vi "Handle RESULT.vi"(8 "error in (no error)":errorcluster, 9 "Message Loop Shift Register Data":T1, 10 "WAMP Message":T16 {"Message Codes" items=["HELLO"=1, "WELCOME"=2, "ABORT"=3, "GOODBYE"=6, "ERROR"=8, "PUBLISH"=16, "PUBLISHED"=17, "SUBSCRIBE"=32, "SUBSCRIBED"=33, "UNSUBSCRIBE"=34, "UNSUBSCRIBED"=35, "EVENT"=36, "CALL"=48, "RESULT"=59, "REGISTER"=64, "REGISTERED"=65, "UNREGISTER"=66, "UNREGISTERED"=67, "INVOCATION"=68, "YIELD"=70]}, 11 "reference":refnum<class "WAMP Client.lvclass">) -> (0 "error out":errorcluster, 1 "Message Loop Shift Register Data (out)":T1, 3 "reference out":refnum<class "WAMP Client.lvclass">)   [LabVIEW 2020, in "wamplv.lvlib" / "WAMP Client.lvclass"]
uses:
  WAMP Client.lvclass
  TypeDef/WAMP Received Message.ctl
  TypeDef/WAMP Message Codes.ctl
  TypeDef/Message Loop Shift Reg Data.ctl
  TypeDef/REGISTER Request Data.ctl
  TypeDef/Success or error.ctl
  API/TypeDefs/Combined error.ctl
  API/TypeDefs/WAMP error.ctl
  API/TypeDefs/Invocation payload.ctl
  TypeDef/Publish Requests Map.ctl
  TypeDef/PUBLISH Request Data.ctl
  TypeDef/PUBLISH Result.ctl
  TypeDef/Endpoint Data.ctl
  TypeDef/CALL Request Map.ctl
  TypeDef/CALL Request Data.ctl
  API/TypeDefs/RESULT Payload.ctl
  TypeDef/SUBSCRIBE Requests Map.ctl
  TypeDef/SUBSCRIBE Request Data.ctl
  TypeDef/Subscribe Result.ctl
  TypeDef/Event Payload.ctl
  TypeDef/Subscriptions Map.ctl
  TypeDef/Subscription Details.ctl
  TypeDef/Unsubscribe Requests Map.ctl
  TypeDef/UNSUBSCRIBE Request Data.ctl
  TypeDef/UNSUBSCRIBE Result.ctl
  TypeDef/Unregister requests map.ctl
  TypeDef/Unregister request.ctl
  WAMP Client.lvclass/WAMP Client.ctl
  <vilib>/JDP Science/JSONtext/JSONtext.lvlib
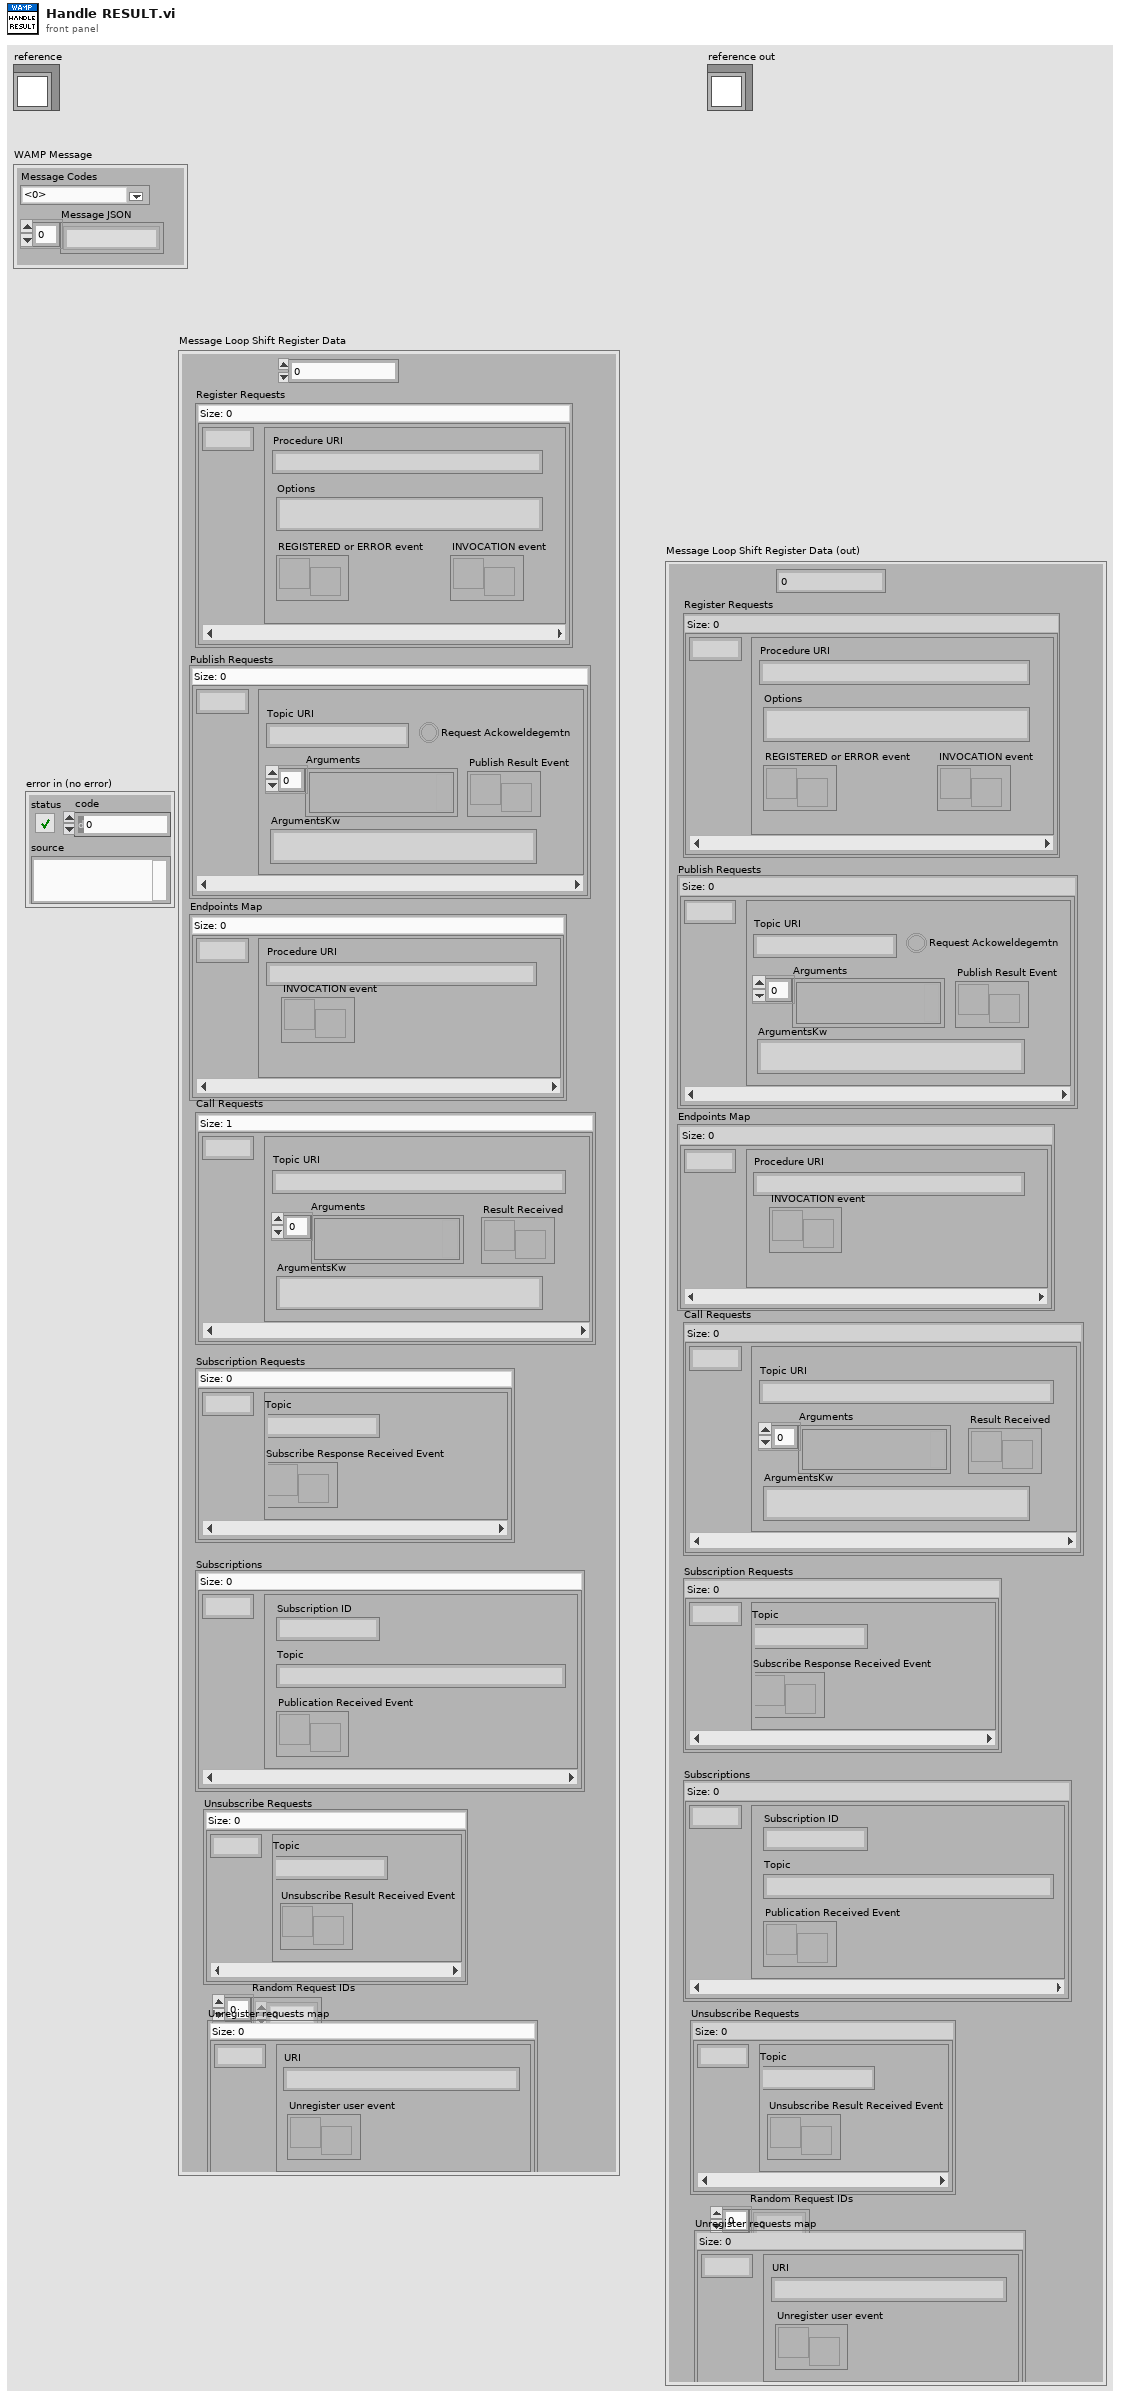
[diagram p1: front panel]
types:
  T1 = typedef "wamplv.lvlib/WAMP Client.lvclass/Message Loop Shift Reg Data.ctl" = cluster{"Last Request ID":u64, "Register Requests":map{u64, T2}, "Publish Requests":T3, "Endpoints Map":map{u64, T5}, "Call Requests":T6, "Subscription Requests":T8, "Subscriptions":T10, "Unsubscribe Requests":T12, "Random Request IDs":u64[], "Unregister requests map":T14}
  T2 = typedef "wamplv.lvlib/WAMP Client.lvclass/REGISTER Request Data.ctl" = cluster{"Procedure URI":string, "Options":string, "REGISTERED or ERROR event":refnum<user-event>, "INVOCATION event":refnum<user-event>}
  T3 = typedef "wamplv.lvlib/WAMP Client.lvclass/Publish Requests Map.ctl" = map{u64, T4}
  T4 = typedef "wamplv.lvlib/WAMP Client.lvclass/PUBLISH Request Data.ctl" = cluster{"Topic URI":string, "Arguments":variant[], "ArgumentsKw":string, "Publish Result Event":refnum<user-event>, "Request Ackoweldegemtn":bool}
  T5 = typedef "wamplv.lvlib/WAMP Client.lvclass/Endpoint Data.ctl" = cluster{"Procedure URI":string, "INVOCATION event":refnum<user-event>}
  T6 = typedef "wamplv.lvlib/WAMP Client.lvclass/CALL Request Map.ctl" = map{u64, T7}
  T7 = typedef "wamplv.lvlib/WAMP Client.lvclass/CALL Request Data.ctl" = cluster{"Topic URI":string, "Arguments":variant[], "ArgumentsKw":string, "Result Received":refnum<user-event>}
  T8 = typedef "wamplv.lvlib/WAMP Client.lvclass/SUBSCRIBE Requests Map.ctl" = map{u64, T9}
  T9 = typedef "wamplv.lvlib/WAMP Client.lvclass/SUBSCRIBE Request Data.ctl" = cluster{"Topic":string, "Subscribe Response Received Event":refnum<user-event>}
  T10 = typedef "wamplv.lvlib/WAMP Client.lvclass/Subscriptions Map.ctl" = map{u64, T11}
  T11 = typedef "wamplv.lvlib/WAMP Client.lvclass/Subscription Details.ctl" = cluster{"Subscription ID":u64, "Topic":string, "Publication Received Event":refnum<user-event>}
  T12 = typedef "wamplv.lvlib/WAMP Client.lvclass/Unsubscribe Requests Map.ctl" = map{u64, T13}
  T13 = typedef "wamplv.lvlib/WAMP Client.lvclass/UNSUBSCRIBE Request Data.ctl" = cluster{"Topic":string, "Unsubscribe Result Received Event":refnum<user-event>}
  T14 = typedef "wamplv.lvlib/WAMP Client.lvclass/Unregister requests map.ctl" = map{u64, T15}
  T15 = typedef "wamplv.lvlib/WAMP Client.lvclass/Unregister request.ctl" = cluster{"URI":string, "Unregister user event":refnum<user-event>}
  T16 = typedef "wamplv.lvlib/WAMP Client.lvclass/WAMP Received Message.ctl" = cluster{"Message JSON":string[], "Message Codes":T17}
  T17 = typedef "wamplv.lvlib/WAMP Client.lvclass/WAMP Message Codes.ctl" = u16
  T18 = typedef "wamplv.lvlib/WAMP Client.lvclass/RESULT Payload.ctl" = cluster{"Arguments Payload":string[], "ArgumentKw Payload":string, "Topic":string, "Success?":bool, "Combined Error":T19}
  T19 = typedef "wamplv.lvlib/WAMP Client.lvclass/Combined error.ctl" = cluster{"Error?":bool, "WAMP Error":T20, "Error":errorcluster}
  T20 = typedef "wamplv.lvlib/WAMP Client.lvclass/WAMP error.ctl" = cluster{"Details":string, "ArgumentKw Payload":string, "Error?":bool, "Error URI":string, "Arguments Payload":string[]}
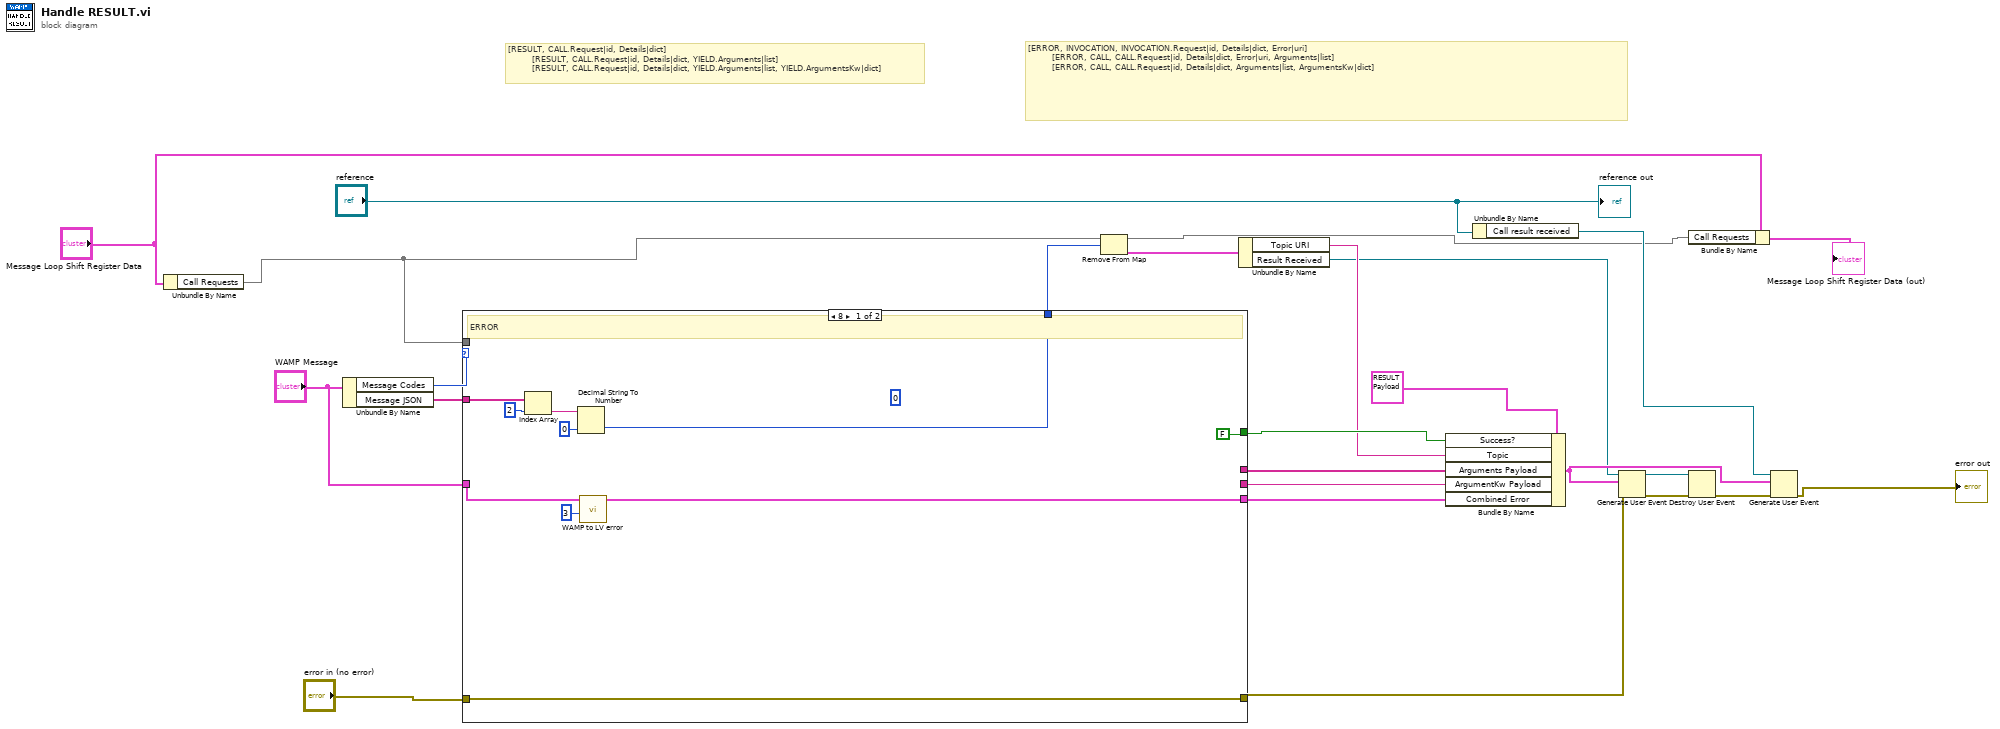
[diagram p0: block diagram]
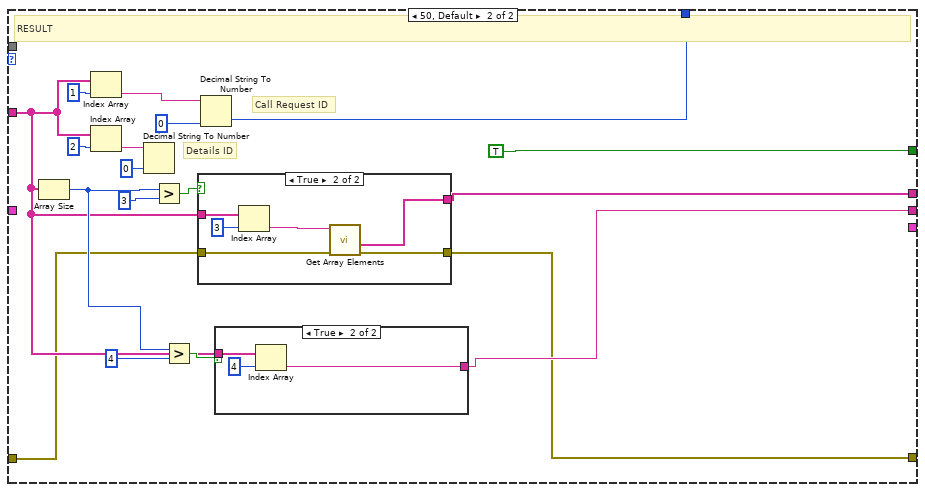
[diagram p2: hidden frame]
diagram:
  # "[ERROR, INVOCATION, INVOCATION.Request|id, Details|dict, Error|uri]\n        [ERROR, CALL, CALL.Request|id, Details|dict, Error|uri, Arguments|list]\n        [ERROR, CALL, CALL.Request|id, Details|dict, Arguments|list, ArgumentsKw|dict]"
  # "[RESULT, CALL.Request|id, Details|dict]\n        [RESULT, CALL.Request|id, Details|dict, YIELD.Arguments|list]\n        [RESULT, CALL.Request|id, Details|dict, YIELD.Arguments|list, YIELD.ArgumentsKw|dict]"
  n1 = Unbundle By Name("Message Loop Shift Register Data") -> ("Call Requests"=w7:T6)
  n2 = Unbundle By Name("WAMP Message") -> ("Message Codes"=w22:T17, "Message JSON"=w21:string[])
  n3 = case shown="8" w22 {
    tunnel: w21 -> [w31 w40]
    tunnel: [w32 w37] -> w20
    tunnel: "error in (no error)" -> [w27 w39]
    tunnel: [w27 w38] -> w23
    tunnel: [FALSE ("Success?") TRUE ("Success?")] -> w24
    tunnel: w7 -> [_ _]
    tunnel: [_ w42] -> w15
    tunnel: [_ w41] -> w14
    tunnel: "WAMP Message" -> [w29 _]
    tunnel: [w26 _] -> w1
    frame 8 {
      (unwired) 0
      # "ERROR"
      n4 = Index Array(array=w31, index=2) -> (element=w34:string)
      n5 = Decimal String To Number(string=w34, default (0L)=u64 0 ("default (0 I32)")) -> (number=w32:u64)  [unwired: 1 in, 1 out]
      n6 = call "WAMP to LV error.vi"("Details Index"=u32 3, "WAMP Message"=w29) -> ("Combined Error"=w26:T19)  [unwired: 7 in, 2 out]
    }
    frame 50, Default {
      # "Call Request ID"
      # "Details ID"
      # "RESULT"
      n7 = Array Size(array=w40) -> (size(s)=w43:i32)
      n8 = Index Array(array=w40, index=1) -> (element=w49:string)
      n9 = Index Array(array=w40, index=2) -> (element=w52:string)
      n10 = Decimal String To Number(string=w52, default (0L)=u32 0) -> ()  [unwired: 1 in, 2 out]
      n11 = Greater?(x=w43, y=3) -> (0:w36:bool)
      n12 = Greater?(x=w43, y=4) -> (0:w44:bool)
      n13 = case shown="True" w36 {
        tunnel: [_ w62] -> w42
        tunnel: [w57 w61] -> w38
        tunnel: w40 -> [_ w60]
        tunnel: w39 -> [w57 w58]
        frame False {
        }
        frame True {
          n14 = Index Array(array=w60, index=3) -> (element=w59:string)
          n15 = call <vilib>:"Get Array Elements.vi"("error in (no error)"=w58, "JSON"=w59) -> ("error out"=w61:errorcluster, "<JSON>"=w62:string[])  [unwired: 7 in, 1 out]
        }
      }
      n16 = Decimal String To Number(string=w49, default (0L)=u32 0) -> (number=w37:u32)  [unwired: 1 in, 1 out]
      n17 = case shown="True" w44 {
        tunnel: [_ w55] -> w41
        tunnel: w40 -> [_ w54]
        frame False {
        }
        frame True {
          n18 = Index Array(array=w54, index=4) -> (element=w55:string)
        }
      }
    }
  }
  n19 = Remove From Map(10:w20, 11:w7) -> (1:w19:T7, 3:w3:T6)  [unwired: 1 out]
  n20 = Unbundle By Name(w19) -> ("Topic URI"=w13:string, "Result Received"=w6:refnum<user-event>)
  n21 = Bundle By Name(cluster=T18 {"Arguments Payload"=[], "ArgumentKw Payload"="", "Topic"="", "Success?"=FALSE, "Combined Error"={"Error?"=FALSE, "WAMP Error"={"Details"="{}", "ArgumentKw Payload"="", "Error?"=FALSE, "Error URI"="", "Arguments Payload"=[]}, "Error"={"status"=FALSE, "code"=0, "source"=""}}} ("RESULT Payload"), "Success?"=w24, "Topic"=w13, "Arguments Payload"=w15, "ArgumentKw Payload"=w14, "Combined Error"=w1) -> (w11:T18)
  n22 = Unbundle By Name("reference") -> ("Call result received"=w10:refnum<user-event>)
  n23 = Generate User Event(user event=w6, event data cluster=w11, error in=w23) -> (user event out=w17:refnum<user-event>, error out=w18:errorcluster)  [unwired: 1 in]
  n24 = Bundle By Name(cluster="Message Loop Shift Register Data", "Call Requests"=w3) -> (→"Message Loop Shift Register Data (out)":T1)
  n25 = Destroy User Event(user event=w17, error in=w18) -> (error out=w9:errorcluster)
  n26 = Generate User Event(user event=w10, event data cluster=w11, error in=w9) -> (error out=→"error out":errorcluster)  [unwired: 1 in, 1 out]
  "reference out" <- "reference"
